vi "TTLReceive.vi"(0 "channel":u16=1 min=1 max=8, 7 "socket in":refnum<class "zmq_socket.lvclass">, 11 "error in":errorcluster) -> (6 "new TTL":bool, 8 "socket out":refnum<class "zmq_socket.lvclass">, 12 "event on":bool, 13 "timestamp":i64, 14 "metadata":string, 15 "error out":errorcluster)   [LabVIEW 2017]
doc: "Attemts to receive one TTL event (non-blocking). If no event is present, then the output \"timeout?\" is true. Otherwise, \"timeout?\" is false and unless an error occurs (such as receiving an event that is not in the TTL format), the other outputs contain the event data."
uses:
  <vilib>/addons/zeromq/zmq_socket.lvclass
  EventBaseType.ctl
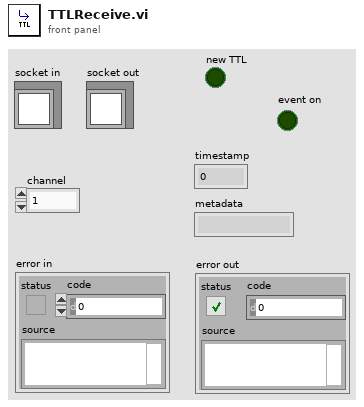
[diagram p1: front panel]
types:
  T1 = enum16{"big-endian, network order", "native, host order", "little-endian"}
  T2 = typedef "EventBaseType.ctl" = enum16{"SYSTEM_EVENT", "PROCESSOR_EVENT", "SPIKE_EVENT"}
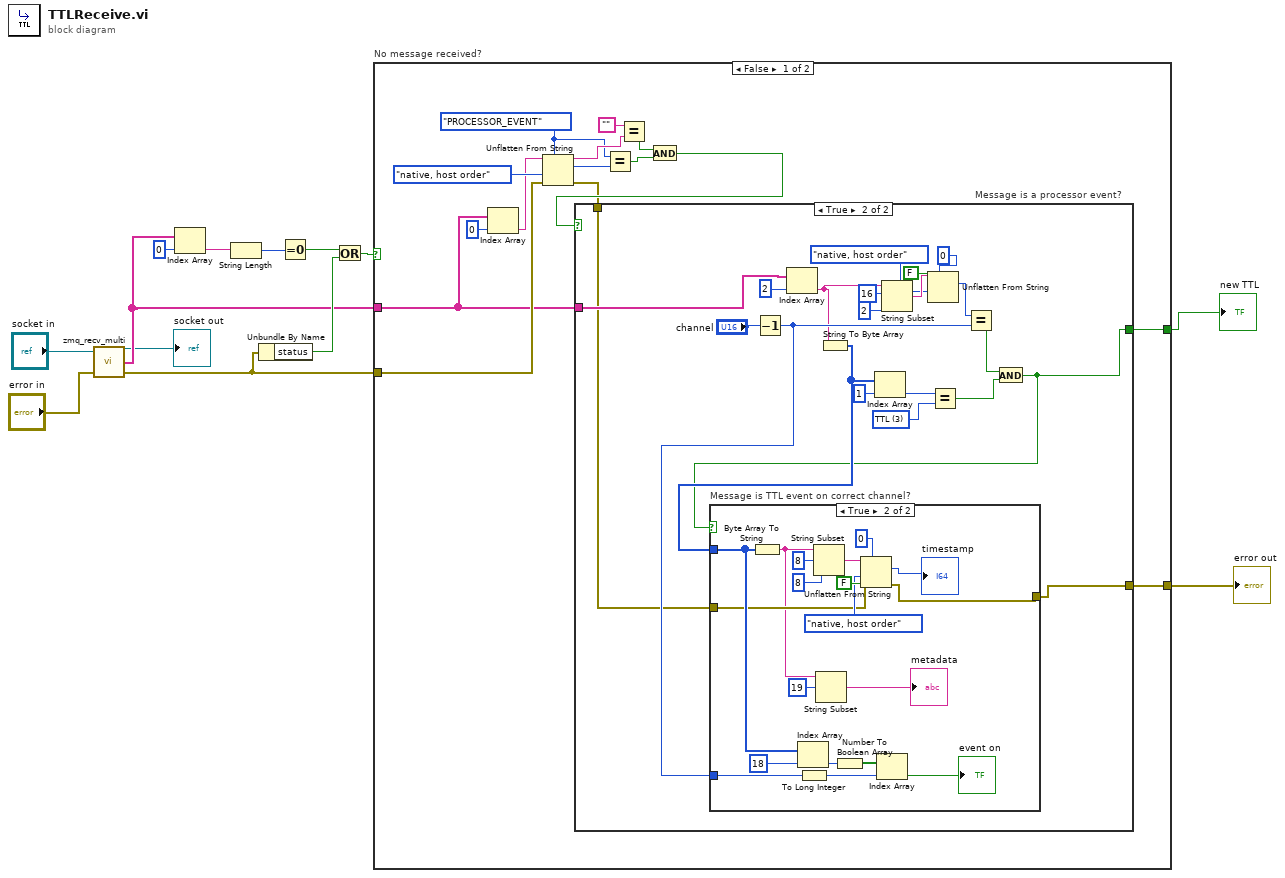
[diagram p0: block diagram]
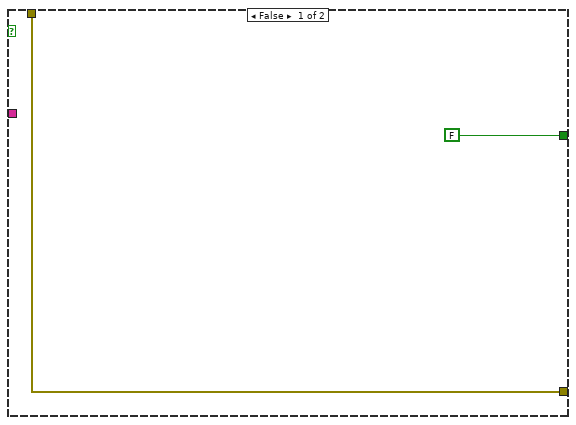
[diagram p2: hidden frame]
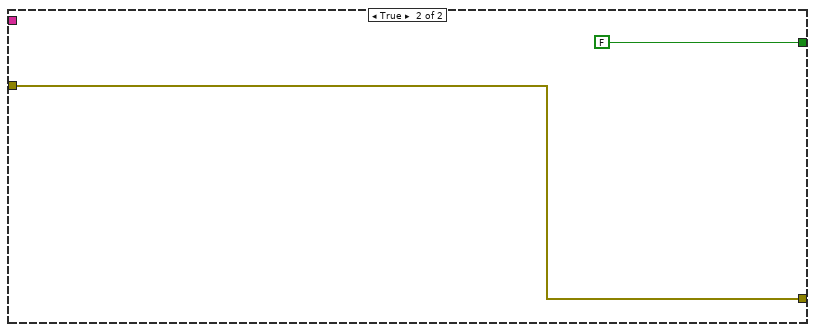
[diagram p4: hidden frame]
diagram:
  n1 = call <vilib>:"zmq_recv_multi.vi"("error in"="error in", "socket in"="socket in") -> ("error out"=w7:errorcluster, "parts"=w2:string[], "socket out"=→"socket out":refnum<class "zmq_socket.lvclass">)  [unwired: 1 in]
  n2 = Index Array(array=w2, index=0) -> (element=w4:string)
  n3 = String Length(string=w4) -> (length=w3:i32)
  n4 = Unbundle By Name(w7) -> ("status"=w10:bool)
  n5 = Equal To 0?(x=w3) -> (x = 0?=w9:bool)
  n6 = Or(x=w9, y=w10) -> (x .or. y?=w11:bool)
  n7 = case "No message received?" shown="False" w11 {
    tunnel: w7 -> [w15 w73]
    tunnel: [w28 w73] -> w13
    tunnel: [w19 FALSE] -> w12
    tunnel: w2 -> [w14 _]
    frame False {
      w18 = EventBaseType."PROCESSOR_EVENT" ("Event base type")
      n8 = Index Array(array=w14, index=0) -> (element=w16:string)
      n9 = Unflatten From String(type=w18, binary string=w16, byte order (0:big-endian, network order)=T1."native, host order", error in (no error)=w15) -> (rest of the binary string=w24:string, value=w26:T2, error out=w20:errorcluster)  [unwired: 1 in]
      n10 = Equal?(x=w18, y=w26) -> (x = y?=w22:bool)
      n11 = Equal?(x="", y=w24) -> (x = y?=w23:bool)
      n12 = And(x=w23, y=w22) -> (x .and. y?=w21:bool)
      n13 = case "Message is a processor event?" shown="True" w21 {
        tunnel: [w30 w41] -> w28
        tunnel: w20 -> [w30 w31]
        tunnel: [FALSE w43] -> w19
        tunnel: w14 -> [_ w32]
        frame False {
        }
        frame True {
          w46 = u8 3 items=["TTL"=3, "TEXT"=5, "INT8_ARRAY"=10, "UINT8_ARRAY"=11, "INT16_ARRAY"=12, "UINT16_ARRAY"=13, "INT32_ARRAY"=14, "UINT32_ARRAY"=15, "INT64_ARRAY"=16, "UINT64_ARRAY"=17, "FLOAT_ARRAY"=18, "DOUBLE_ARRAY"=19, "INVALID"=20]
          n14 = Decrement(x="channel") -> (x-1=w42:u16)
          n15 = Index Array(array=w32, index=2) -> (element=w38:string)
          n16 = String To Byte Array(string=w38) -> (unsigned byte array=w49:u8[])
          n17 = Index Array(array=w49, index=1) -> (element=w47:u8)
          n18 = String Subset(string=w38, offset (0)=16, length (rest)=2 ("length (rest)")) -> (substring=w37:string)
          n19 = Unflatten From String(type=u16 0, binary string=w37, data includes array or string size? (T)=FALSE, byte order (0:big-endian, network order)=T1."native, host order") -> (value=w33:u16)  [unwired: 1 in, 2 out]
          n20 = Equal?(x=w47, y=w46) -> (x = y?=w45:bool)
          n21 = Equal?(x=w33, y=w42) -> (x = y?=w44:bool)
          n22 = And(x=w44, y=w45) -> (x .and. y?=w43:bool)
          n23 = case "Message is TTL event on correct channel?" shown="True" w43 {
            tunnel: w49 -> [_ w67]
            tunnel: w42 -> [_ w54]
            tunnel: w31 -> [w52 w59]
            tunnel: [w52 w58] -> w41
            frame False {
            }
            frame True {
              n24 = Byte Array To String(unsigned byte array=w67) -> (string=w57:string)
              n25 = Index Array(array=w67, index=18) -> (element=w70:u8)
              n26 = To Long Integer(number=w54) -> (32bit integer=w53:i32)
              n27 = String Subset(string=w57, offset (0)=8, length (rest)=8 ("length (rest)")) -> (substring=w64:string)
              n28 = String Subset(string=w57, offset (0)=19) -> (substring=→"metadata":string)  [unwired: 1 in]
              n29 = Number To Boolean Array(number=w70) -> (Boolean array=w69:bool[])
              n30 = Unflatten From String(type=i64 0, binary string=w64, data includes array or string size? (T)=FALSE, byte order (0:big-endian, network order)=T1."native, host order", error in (no error)=w59) -> (value=→"timestamp":i64, error out=w58:errorcluster)  [unwired: 1 out]
              n31 = Index Array(array=w69, index=w53) -> (element=→"event on":bool)
            }
          }
        }
      }
    }
    frame True {
    }
  }
  "error out" <- w13
  "new TTL" <- w12
